vi "sedSpectrometer_getEvent_rejectedCommand.vi"(8 "error in (no error)":errorcluster, 11 "logevent_rejectedCommand_Ctl":T1) -> (0 "error out":errorcluster, 2 "function return":i32, 3 "logevent_rejectedCommand_Ctl out":T1)   [LabVIEW 2016, in "SALLV_sedSpectrometer.lvlib"]
doc: "int sedSpectrometer_shm_getEvent_rejectedCommandLV(sedSpectrometer_logevent_rejectedCommandLV *logevent_rejectedCommand_Ctl );"
uses:
  SALLV_sedSpectrometer.lvlib
  DataTypes/logevent_rejectedCommand.ctl
  SALLV_sedSpectrometer.so
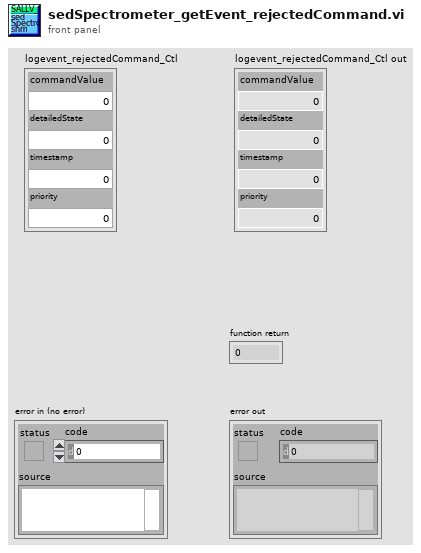
[diagram p1: front panel]
types:
  T1 = typedef "SALLV_sedSpectrometer.lvlib/logevent_rejectedCommand.ctl" = cluster{"commandValue":u16, "detailedState":u16, "timestamp":dbl, "priority":i32}
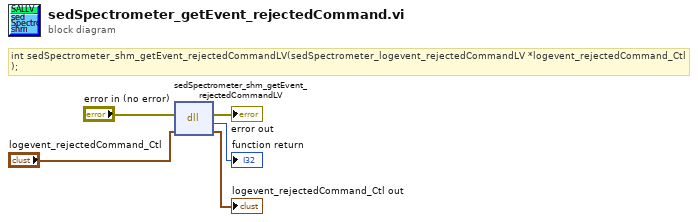
[diagram p0: block diagram]
diagram:
  # "int sedSpectrometer_shm_getEvent_rejectedCommandLV(sedSpectrometer_logevent_rejectedCommandLV *logevent_rejectedCommand_Ctl );"
  n1 = dll-call lib="home/harini/TCS/ts_sallv_sedSpectrometer_371/SALLV_sedSpectrometer.*" fn="sedSpectrometer_shm_getEvent_rejectedCommandLV"(error in="error in (no error)", "logevent_rejectedCommand_Ctl"="logevent_rejectedCommand_Ctl") -> (error out=→"error out":errorcluster, →"function return":i32, "logevent_rejectedCommand_Ctl"=→"logevent_rejectedCommand_Ctl out":T1)  [unwired: 2 in, 1 out]
